vi "Run VI.vi"(7 "불리언":bool, 8 "에러 입력(에러 없음)":errorcluster, 9 "서브패널 입력":refnum<vi>, 10 "VI 참조 번호 입력":refnum<vi>) -> (0 "에러 출력":errorcluster, 3 "VI 출력":refnum<vi>)   [LabVIEW 2023]
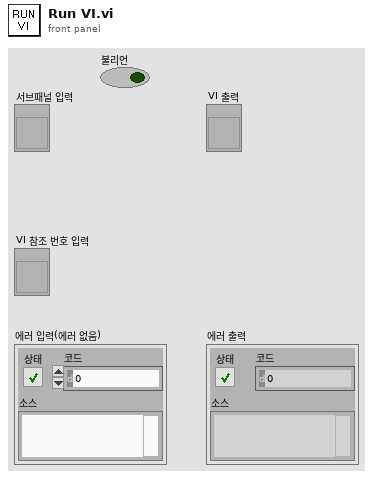
[diagram p1: front panel]
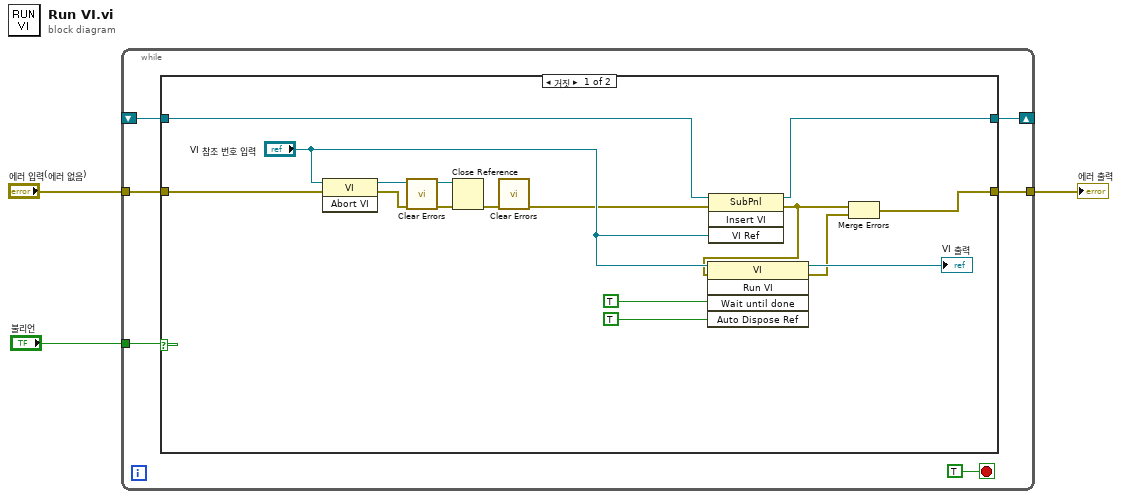
[diagram p0: block diagram]
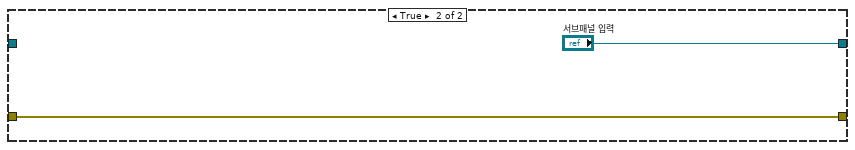
[diagram p2: hidden frame]
diagram:
  n1 = while {
    shift-right: [w8] -> _
    shift-left: _ -> [w7]
    tunnel: "에러 입력(에러 없음)" -> [w6]
    tunnel: [w5] -> w2
    tunnel: "불리언" -> [w4]
    stop <- TRUE stop-if-true
    n2 = case shown="거짓" w4 {
      tunnel: [w11 "서브패널 입력"] -> w8
      tunnel: w7 -> [w21 _]
      tunnel: w6 -> [w19 w25]
      tunnel: [w18 w25] -> w5
      frame False {
        n3 = invoke class="VI" method="Abort VI"(reference="VI 참조 번호 입력", error in=w19) -> (reference out=w14:refnum<vi>, error out=w15:errorcluster)  [unwired: 1 in, 1 out]
        n4 = call <vilib>:"Clear Errors.vi"("error in (no error)"=w15) -> ("error out"=w16:errorcluster)  [unwired: 5 in, 1 out]
        n5 = Close Reference(reference=w14, error in (no error)=w16) -> (error out=w17:errorcluster)
        n6 = call <vilib>:"Clear Errors.vi"("error in (no error)"=w17) -> ("error out"=w12:errorcluster)  [unwired: 5 in, 1 out]
        n7 = invoke on="인보크 노드" class="SubPnl" method="Insert VI"(reference=w21, error in=w12, "VI Ref"="VI 참조 번호 입력") -> (reference out=w11:refnum<vi>, error out=w10:errorcluster)  [unwired: 1 in, 2 out]
        n8 = invoke class="VI" method="Run VI"(reference="VI 참조 번호 입력", error in=w10, "Wait until done"=TRUE ("Wait Until Done"), "Auto Dispose Ref"=TRUE ("Auto Dispose Reference")) -> (reference out=→"VI 출력":refnum<vi>, error out=w20:errorcluster)  [unwired: 1 in, 3 out]
        n9 = Merge Errors(w10, w20) -> (w18:errorcluster)
      }
      frame True {
      }
    }
  }
  "에러 출력" <- w2
